vi "Mosaic status.vi"(7 "Actions":T2=enum."Clear", 8 "Error In":errorcluster, 10 "Status In":bool, 11 "Mosaic status in":T1) -> (0 "Error Out":errorcluster, 2 "Status Out":bool, 3 "Mosaic status out":T1)   [LabVIEW 2018]
uses:
  Controls/FGV Actions.ctl
  Controls/Go Scan Actions.ctl
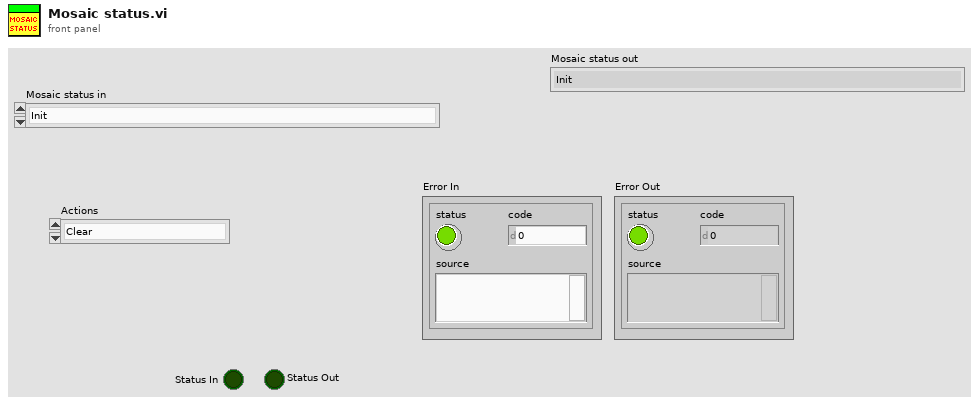
[diagram p1: front panel]
types:
  T1 = typedef "Go Scan Actions.ctl" = enum16{"Init", "Init Scan Head", "Init Table Stage", "Init Vibratome", "Generate Mosaic", "Go Image Home", "Go Mosaic", "Acquire Image", "Go Vibratome", "Slice", "Finished"}
  T2 = typedef "FGV Actions.ctl" = enum16{"Init", "Set", "Get", "Clear"}
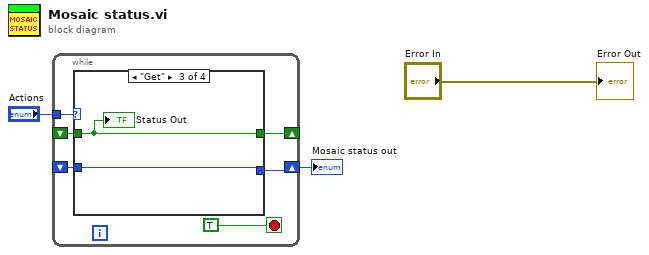
[diagram p0: block diagram]
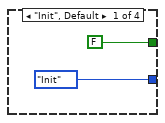
[diagram p2: hidden frame]
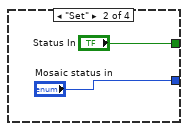
[diagram p3: hidden frame]
diagram:
  n1 = while {
    tunnel: "Actions" -> [w8]
    shift-right: [w7] -> _
    shift-left: _ -> [w6]
    shift-right: [w4] -> w1
    shift-left: _ -> [w5]
    stop <- TRUE stop-if-true
    n2 = case shown="\"Get\"" w8 {
      tunnel: [FALSE "Status In" w15 _] -> w7
      tunnel: w6 -> [_ _ w15 _]
      tunnel: w5 -> [_ _ w14 _]
      tunnel: [Go_Scan_Actions."Init" ("Mosaic status in") "Mosaic status in" w14 _] -> w4
      frame "Init", Default {
      }
      frame "Set" {
      }
      frame "Get" {
        "Status Out" <- w15
      }
      frame "Clear" {
      }
    }
  }
  "Mosaic status out" <- w1
  "Error Out" <- "Error In"
